vi "Empty TEMP Folder.vi"(8 "error in (no error)":errorcluster) -> (0 "error out":errorcluster, 2 "TEMP Folder Deleted":bool)   [LabVIEW 2024]
doc: "Stop analysis immediately by stopping python script running. Delete all features found for current image to avoid duplicates in future."
uses:
  <vilib>/Utility/sysdir.llb/System Directory Type.ctl
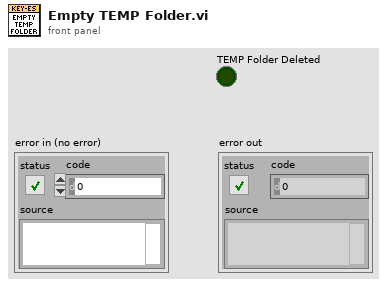
[diagram p1: front panel]
types:
  T1 = typedef "System Directory Type.ctl" = i32
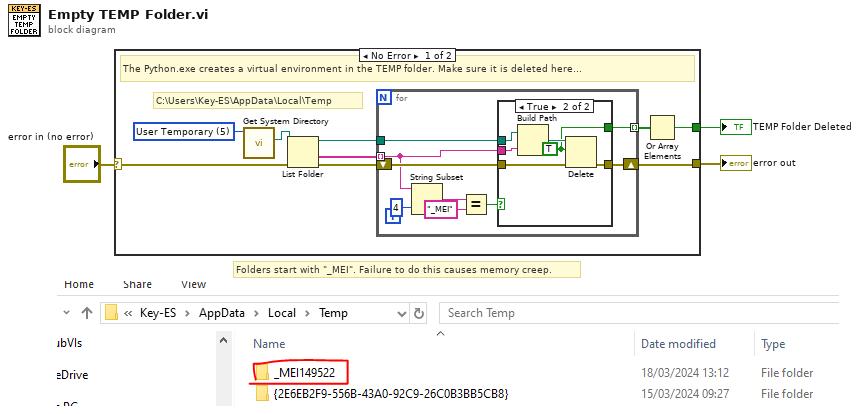
[diagram p0: block diagram]
diagram:
  # "Folders start with \"_MEI\". Failure to do this causes memory creep."
  n1 = case shown="No Error" "error in (no error)" {
    selector: "error in (no error)" -> [w12 w29]
    tunnel: [w6 w29] -> w3
    tunnel: [w4 _] -> w1
    frame No Error {
      w11 = T1 5 items=["User Home"=0, "User Desktop"=1, "User Documents"=2, "User Application Data"=3, "User Preferences"=4, "User Temporary"=5, "Public Documents"=6, "Public Application Data"=7, "Public Preferences"=8, "Public Cache"=13, "System Core Libraries"=9, "System Installed Libraries"=10, "Application Files"=11, "Boot Volume Root"=12] ("system directory type")
      # "C:\\Users\\Key-ES\\AppData\\Local\\Temp"
      # "The Python.exe creates a virtual environment in the TEMP folder. Make sure it is deleted here..."
      n2 = call <vilib>:"Get System Directory.vi"("system directory type"=w11) -> ("system directory"=w10:path)  [unwired: 10 in]
      n3 = List Folder(path=w10, error in=w12) -> (path out=w8:path, folder names=w9:string[], error out=w7:errorcluster)  [unwired: 2 in, 1 out]
      n4 = for {
        tunnel: w9 -> [w14] mode=indexing
        tunnel: w8 -> [w15]
        shift-right: [w16] -> w6
        shift-left: w7 -> [w17]
        tunnel: [w13] -> w5 mode=indexing
        n5 = String Subset(string=w14, length (rest)=4 ("length (rest)")) -> (substring=w21:string)  [unwired: 1 in]
        n6 = Equal?(x=w21, y="_MEI") -> (x = y?=w18:bool)
        n7 = case shown="True" w18 {
          tunnel: w17 -> [w22 w28]
          tunnel: [w22 w27] -> w16
          tunnel: w15 -> [_ w25]
          tunnel: w14 -> [_ w24]
          tunnel: [_ w23] -> w13
          frame False {
          }
          frame True {
            w23 = TRUE ("entire hierarchy (F)")
            n8 = Build Path(base path=w25, name or relative path=w24) -> (appended path=w26:path)
            n9 = Delete(path (use dialog)=w26, entire hierarchy (F)=w23, error in=w28) -> (error out=w27:errorcluster)  [unwired: 2 in, 2 out]
          }
        }
      }
      n10 = Or Array Elements(Boolean array=w5) -> (logical OR=w4:bool)
    }
    frame Error {
    }
  }
  "error out" <- w3
  "TEMP Folder Deleted" <- w1
